vi "DB_Action-DeleteModule.vi"(8 "error in":errorcluster, 10 "Name":string="4032248904914", 11 "路径":path=path "E:/FCT File Share/29_WDML/SO-20969 MSNG/7_Code/3_Software/0_DB_Action/3_Data/WDML.mdb") -> (0 "error out":errorcluster)   [LabVIEW 2015, in "Settings-Style.lvlib"]
uses:
  Settings-Style.lvlib
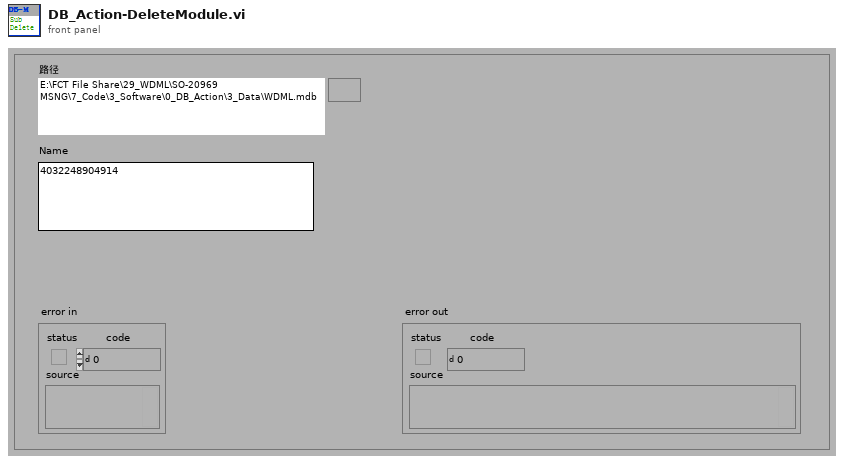
[diagram p1: front panel]
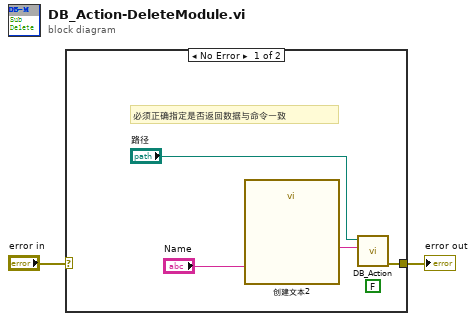
[diagram p0: block diagram]
diagram:
  n1 = case shown="No Error" "error in" {
    selector: "error in" -> [_ w7]
    tunnel: [w3 w7] -> w2
    frame No Error {
      (unwired) FALSE ("Return Data (T)")
      # "必须正确指定是否返回数据与命令一致"
      n2 = call "创建文本2"("Name"="Name") -> ("Result"=w4:string)  [unwired: 13 in, 1 out]
      n3 = call "DB_Action.vi"("Command Text"=w4, "路径"="路径") -> ("error out"=w3:errorcluster)  [unwired: 8 in, 1 out]
    }
    frame Error {
    }
  }
  "error out" <- w2
